vi "dfd_Util I160 Adder.vi"(8 "y160":T1, 11 "x160":T1) -> (3 "x+y160":T1)   [LabVIEW 2017, in "NI_DigFilter_FXP.lvlib"]
uses:
  <vilib>/addons/Digital Filter Design/NI_DigFilter_FXP.lvlib
  <vilib>/addons/Digital Filter Design/_Objects.llb/dfd_Integer I160.ctl
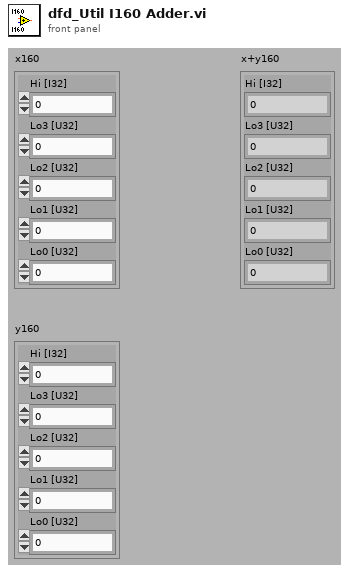
[diagram p1: front panel]
types:
  T1 = typedef "dfd_Integer I160.ctl" = cluster{"Hi [I32]":i32, "Lo3 [U32]":u32, "Lo2 [U32]":u32, "Lo1 [U32]":u32, "Lo0 [U32]":u32}
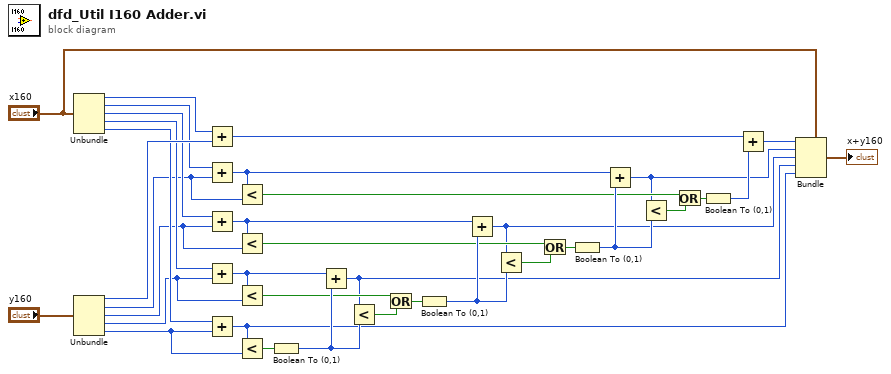
[diagram p0: block diagram]
diagram:
  n1 = Unbundle("x160") -> ("Hi [I32]"=w33:i32, "Lo3 [U32]"=w8:u32, "Lo2 [U32]"=w7:u32, "Lo1 [U32]"=w6:u32, "Lo0 [U32]"=w5:u32)
  n2 = Unbundle("y160") -> ("Hi [I32]"=w32:i32, "Lo3 [U32]"=w4:u32, "Lo2 [U32]"=w3:u32, "Lo1 [U32]"=w2:u32, "Lo0 [U32]"=w1:u32)
  n3 = Add(x=w33, y=w32) -> (x+y=w16:i32)
  n4 = Add(x=w8, y=w4) -> (x+y=w20:u32)
  n5 = Add(x=w7, y=w3) -> (x+y=w25:u32)
  n6 = Add(x=w6, y=w2) -> (x+y=w30:u32)
  n7 = Add(x=w5, y=w1) -> (x+y=w9:u32)
  n8 = Less?(x=w20, y=w4) -> (x < y?=w18:bool)
  n9 = Less?(x=w25, y=w3) -> (x < y?=w23:bool)
  n10 = Less?(x=w30, y=w2) -> (x < y?=w28:bool)
  n11 = Less?(x=w9, y=w1) -> (x < y?=w31:bool)
  n12 = Boolean To (0,1)(Boolean=w31) -> (0, 1=w29:i16)
  n13 = Add(x=w30, y=w29) -> (x+y=w10:u32)
  n14 = Less?(x=w10, y=w29) -> (x < y?=w27:bool)
  n15 = Or(x=w28, y=w27) -> (x .or. y?=w26:bool)
  n16 = Boolean To (0,1)(Boolean=w26) -> (0, 1=w24:i16)
  n17 = Add(x=w25, y=w24) -> (x+y=w11:u32)
  n18 = Less?(x=w11, y=w24) -> (x < y?=w22:bool)
  n19 = Or(x=w23, y=w22) -> (x .or. y?=w21:bool)
  n20 = Boolean To (0,1)(Boolean=w21) -> (0, 1=w19:i16)
  n21 = Add(x=w20, y=w19) -> (x+y=w12:u32)
  n22 = Less?(x=w12, y=w19) -> (x < y?=w17:bool)
  n23 = Or(x=w18, y=w17) -> (x .or. y?=w15:bool)
  n24 = Boolean To (0,1)(Boolean=w15) -> (0, 1=w14:i16)
  n25 = Add(x=w16, y=w14) -> (x+y=w13:i32)
  n26 = Bundle(cluster="x160", "Hi [I32]"=w13, "Lo3 [U32]"=w12, "Lo2 [U32]"=w11, "Lo1 [U32]"=w10, "Lo0 [U32]"=w9) -> (→"x+y160":T1)
